vi "Make freq sweep signal.vi"(0 "stimdurfreqsweep":dbl, 1 "nsamp":dbl, 2 "Output freq (Hz)":dbl, 3 "startfreq":dbl, 4 "endfreq":dbl, 5 "sinamp":dbl, 6 "noiseamp":dbl, 7 "beforefreqsweep":dbl, 8 "hicutoff":dbl, 9 "afterfreqsweep":dbl, 10 "lowcutoff":dbl, 11 "position noise? (or velocity)":bool) -> (14 "Stimulus":T2={"type"=enum."Zero", "sinfreq start"=0.0, "sinfreq end"=0.0, "sinamp start"=0.0, "sinamp end"=0.0, "noise freq lo"=0.0, "noise freq hi"=0.0, "noiseamp start"=0.0, "noiseamp end"=0.0, "stimdur"=0.0, "before dur"=0.0, "after dur"=0.0, "pulse data"={"time"=[], "phase/vel"=[], "dir/shift"=[], "amplitude"=[], "duration"=[]}} {"noise freq hi" min=0.0 step=0.5; "noise freq lo" min=0.0 step=0.5; "noiseamp end" min=0.0 step=0.5; "noiseamp start" min=0.0 step=0.5}, 15 "signal":dbl[](array[numeric]), 16 "noise":dbl[](array[numeric]), 17 "phases":T1)   [LabVIEW 2013]
uses:
  Stimulus.ctl
  Stimulus type.ctl
  Pulse data.ctl
  Phases.ctl
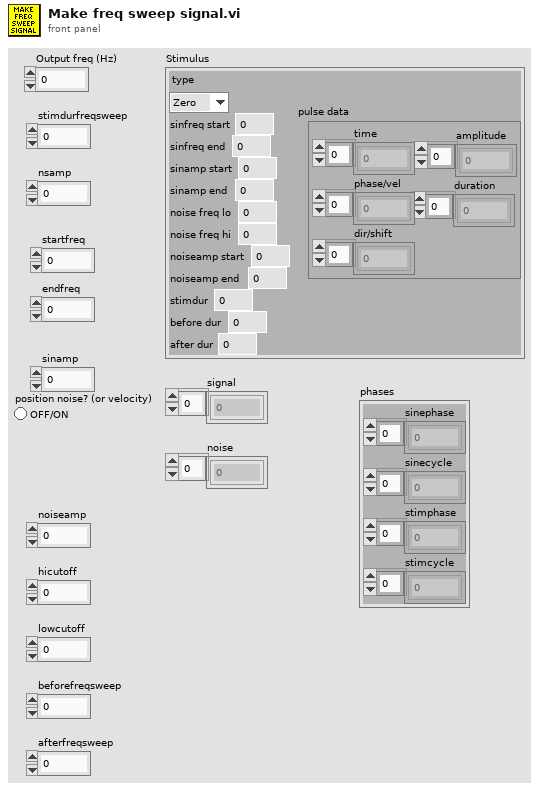
[diagram p1: front panel]
types:
  T1 = typedef "Phases.ctl" = cluster{"sinephase":dbl[], "sinecycle":dbl[], "stimphase":dbl[], "stimcycle":dbl[]}
  T2 = typedef "Stimulus.ctl" = cluster{"type":T3, "sinfreq start":dbl, "sinfreq end":dbl, "sinamp start":dbl, "sinamp end":dbl, "noise freq lo":dbl, "noise freq hi":dbl, "noiseamp start":dbl, "noiseamp end":dbl, "stimdur":dbl, "before dur":dbl, "after dur":dbl, "pulse data":T4}
  T3 = typedef "Stimulus type.ctl" = enum16{"Sine", "Zero", "Frequency sweep", "Two frequency", "Amplitude sweep", "Pulses", "Shifts", "Ramps"}
  T4 = typedef "Pulse data.ctl" = cluster{"time":dbl[], "phase/vel":dbl[], "dir/shift":dbl[], "amplitude":dbl[], "duration":dbl[]}
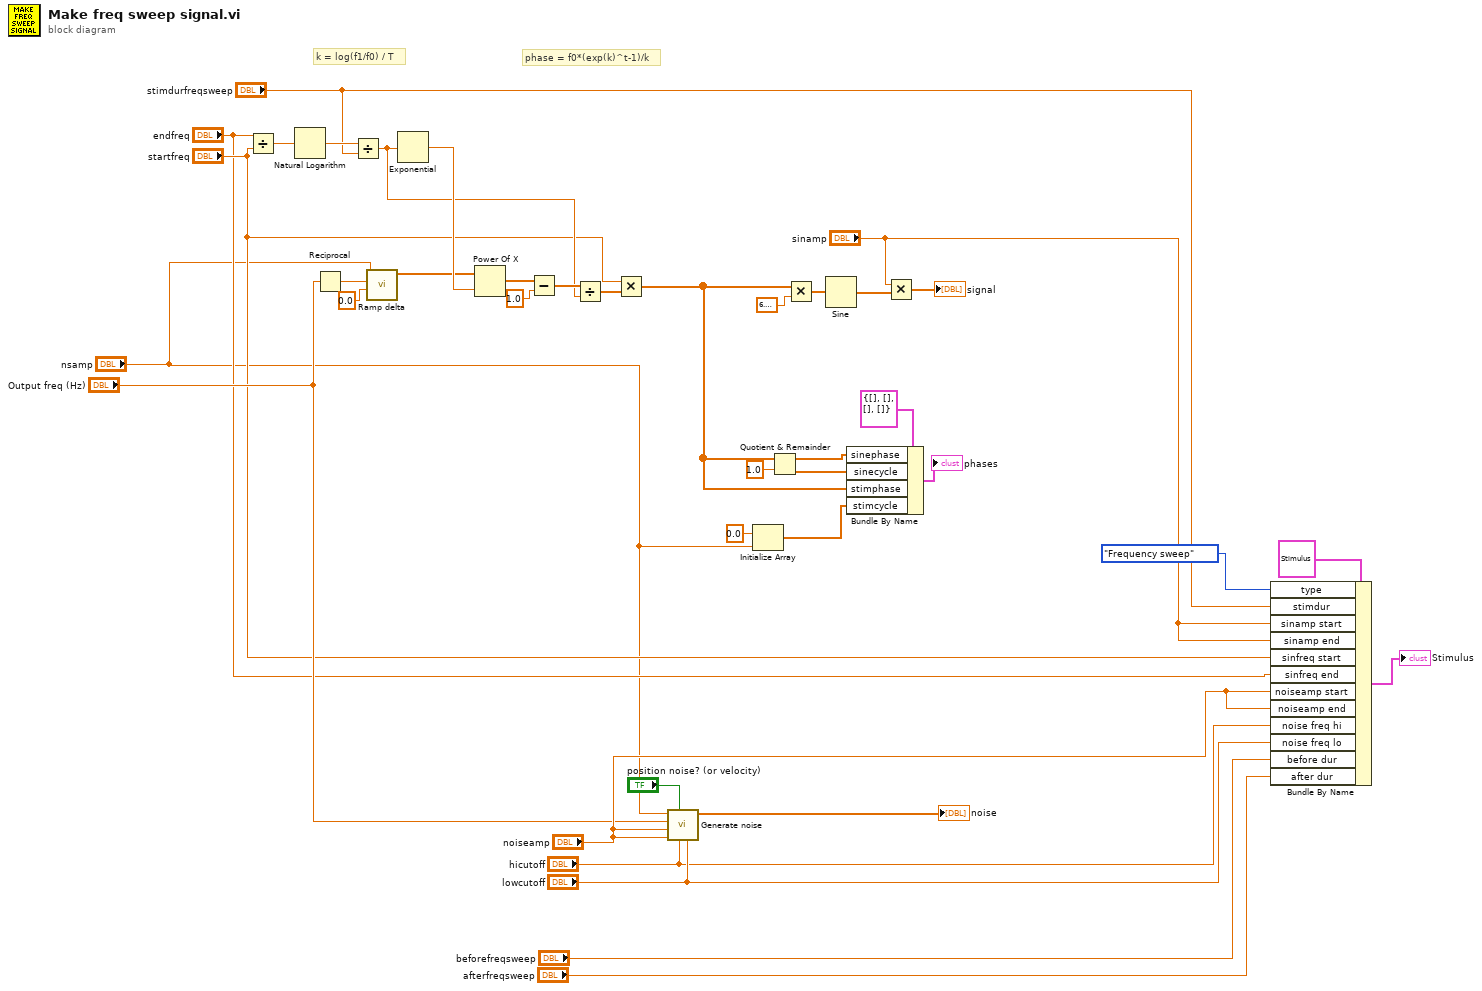
[diagram p0: block diagram]
diagram:
  # "phase = f0*(exp(k)^t-1)/k"
  # "k = log(f1/f0) / T"
  n1 = Divide(x="endfreq", y="startfreq") -> (x/y=w29:dbl)
  n2 = Natural Logarithm(1:w29) -> (0:w28:dbl)
  n3 = Reciprocal(x="Output freq (Hz)") -> (1/x=w32:dbl)
  n4 = Divide(x=w28, y="stimdurfreqsweep") -> (x/y=w22:dbl)
  n5 = call "Ramp delta.vi"("start"=0.0, "delta"=w32, "samples"="nsamp") -> ("ramp signal"=w9:dbl[])  [unwired: 7 in, 1 out]
  n6 = Exponential(1:w22) -> (0:w26:dbl)
  n7 = Power Of X(1:w26, 2:w9) -> (0:w25:dbl[])
  n8 = Subtract(x=w25, y=1.0 ("start")) -> (x-y=w23:dbl[])
  n9 = Divide(x=w23, y=w22) -> (x/y=w21:dbl[])
  n10 = Multiply(x="startfreq", y=w21) -> (x*y=w7:dbl[])
  n11 = call "Generate noise.vi"("lo cutoff"="lowcutoff", "hi cutoff"="hicutoff", "position noise? (or velocity)"="position noise? (or velocity)", "start amplitude"="noiseamp", "end amplitude"="noiseamp", "sampling freq"="Output freq (Hz)", "samples"="nsamp") -> ("noise"=→"noise":dbl[])  [unwired: 4 in]
  n12 = Initialize Array(0.0 ("element"), "nsamp") -> (w4:dbl[])
  n13 = Quotient & Remainder(x=w7, y=1.0 ("start")) -> (x-y*floor(x/y)=w8:dbl[], floor(x/y)=w14:dbl[])
  n14 = Multiply(x=w7, y=6.283185307179586) -> (x*y=w19:dbl[])
  n15 = Sine(x=w19) -> (sin(x)=w18:dbl[])
  n16 = Bundle By Name(cluster=T1 {"sinephase"=[], "sinecycle"=[], "stimphase"=[], "stimcycle"=[]} ("phases"), "sinephase"=w8, "sinecycle"=w14, "stimphase"=w7, "stimcycle"=w4) -> (→"phases":T1)
  n17 = Multiply(x="sinamp", y=w18) -> (x*y=→"signal":dbl[])
  n18 = Bundle By Name(cluster=T2 {"type"=enum."Zero", "sinfreq start"=0.0, "sinfreq end"=0.0, "sinamp start"=0.0, "sinamp end"=0.0, "noise freq lo"=0.0, "noise freq hi"=0.0, "noiseamp start"=0.0, "noiseamp end"=0.0, "stimdur"=0.0, "before dur"=0.0, "after dur"=0.0, "pulse data"={"time"=[], "phase/vel"=[], "dir/shift"=[], "amplitude"=[], "duration"=[]}} ("Stimulus 2"), "type"=Stimulus_type."Frequency sweep", "stimdur"="stimdurfreqsweep", "sinamp start"="sinamp", "sinamp end"="sinamp", "sinfreq start"="startfreq", "sinfreq end"="endfreq", "noiseamp start"="noiseamp", "noiseamp end"="noiseamp", "noise freq hi"="hicutoff", "noise freq lo"="lowcutoff", "before dur"="beforefreqsweep", "after dur"="afterfreqsweep") -> (→"Stimulus":T2)
